vi "test_assert_not_string.vi"   [LabVIEW 2021]
uses:
  43c10be0-616b-3fbd-cdcc-12529203e63f.vi
  52cd2680-c682-3fbb-9ee2-5137eaa1e33f.vi
  7129dad8-c207-3fd8-386f-c49903dfdc3f.vi
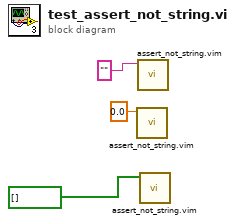
[diagram p0: block diagram]
diagram:
  n1 = call "assert_not_string.vim"("Numeric"=0.0) -> ()  [unwired: 10 in, 1 out]
  n2 = call "assert_not_string.vim"("Numeric"="") -> ()  [unwired: 10 in, 1 out]
  n3 = call "assert_not_string.vim"("Numeric"=bool[] []) -> ()  [unwired: 10 in, 1 out]
